vi "Periodic Tasks.vi"(8 "error in":errorcluster) -> ()   [LabVIEW 2015]
doc: "This VI runs in parallel to other tasks. It can contain as many user-defined periodic loops as you need. These can carry out PID or other sorts of timed response."
uses:
  <vilib>/Rock Robotics/WPI/Solenoid/WPI_SolenoidValue.ctl
  <vilib>/Rock Robotics/WPI/Utilities/WPI_GetSetVariantRefNum.vi
  Robot Global Data.vi
  <vilib>/Rock Robotics/WPI/Solenoid/WPI_SolenoidSetEnum.vi
  <vilib>/Rock Robotics/Network Tables/NT Write Boolean.vi
  <vilib>/Rock Robotics/Network Tables/NT Read Boolean.vi
  <vilib>/Rock Robotics/Network Tables/NT Read Number.vi
  <vilib>/addons/control/pid/pid.llb/PID (DBL).vi
  <vilib>/addons/control/pid/NI_PID_pid.lvlib
panel:
  out "Shoot Speed":dbl
  in  "Aiming Correction":dbl=-0.22
  out "Shoot Motor Output bottom 2":dbl
  out "Shoot Motor Output top 2":dbl
  out "Ball in Robot":bool
  out "Joystick Buttons":bool[](array[boolean])
  out "Joystick Axes":dbl[](array[numeric])
  out "RD before":bool
  out "RU before":bool
  out "R after":bool
  out "L after":bool
  out "LD before":bool
  out "LU before":bool
  out "Intake Mode":bool
  out "Low Mode":bool
  out "Shoot Sequence Position":dbl
  in  "Forklift Method":bool
  in  "Manual Shoot Speed":dbl=0.9
  out "Closed Loop Error":dbl
  out "Sensor Position":dbl
  in  "Expected position":dbl
  in  "Intake Speed":dbl=1.0
  out "Shoot Motor Output bottom":dbl
  out "Shoot Motor Output top":dbl
  in  "Aiming Speed":dbl(slide)=0.3 scale=0.0..1.0
  # "0 = Wait for trigger\n1 = Speed up and aim\n2 = Spin Rollers\n3 = Stop motors"
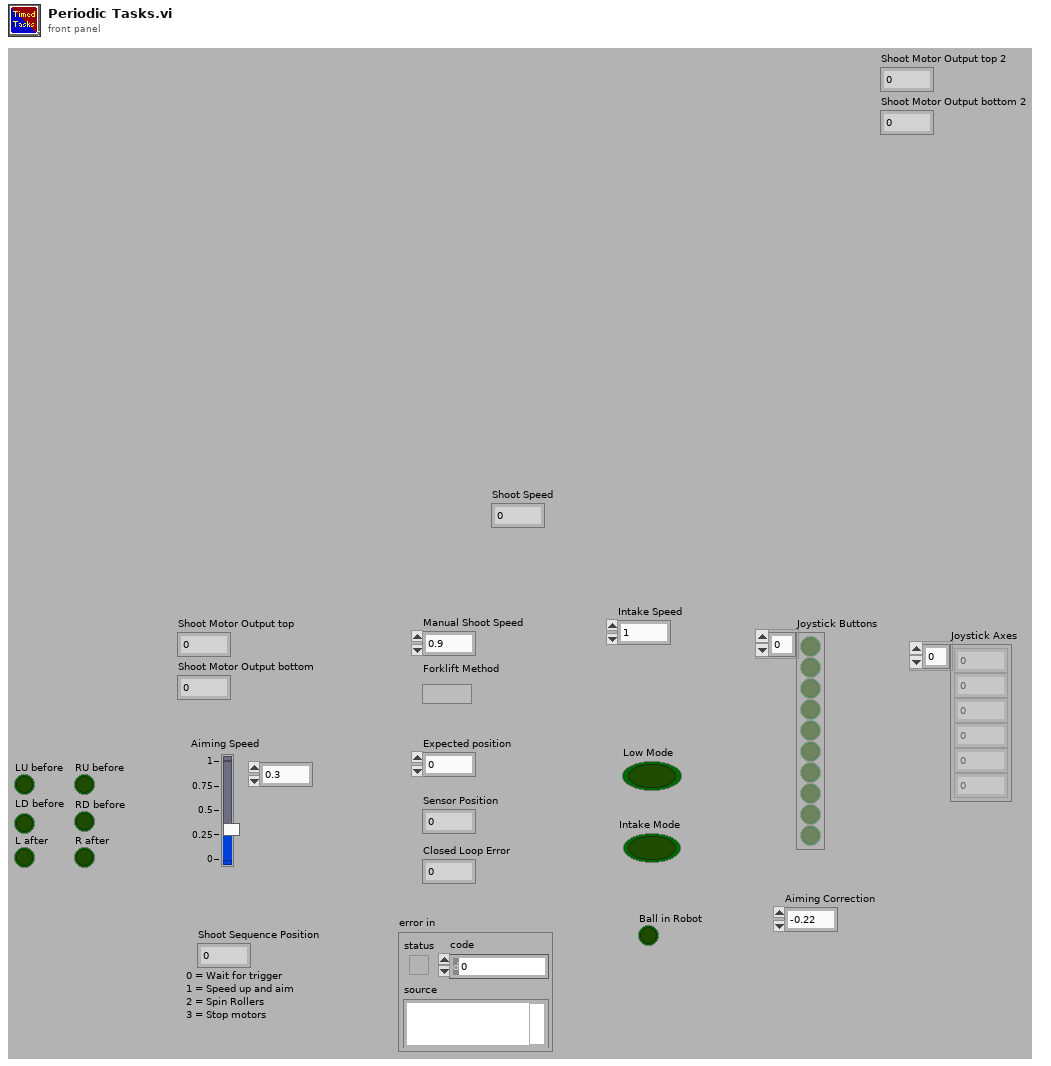
[diagram p1: front panel]
types:
  T1 = typedef "WPI_SolenoidDevRef.ctl" = cluster{"DevStatus":errorcluster, "Pneumatics Control Module":u8, "Forward Solenoid Channel":T2, "Reverse Solenoid Channel":T2}
  T2 = typedef "WPI_SolenoidChannel.ctl" = enum8{"Solenoid 0", "Solenoid 1", "Solenoid 2", "Solenoid 3", "Solenoid 4", "Solenoid 5", "Solenoid 6", "Solenoid 7", "Invalid"}
  T3 = typedef "WPI_JoystickDevRef.ctl" = cluster{"Device":T4}
  T4 = typedef "WPI_JoystickDeviceEnum.ctl" = enum16{"USB 0", "USB 1", "USB 2", "USB 3", "USB 4", "USB 5"}
  T5 = typedef "WPI_RobotDriveDevRef.ctl" = cluster{"DevStatus":errorcluster, "Motors[]":T6[], "Square Inputs":bool, "Max Output":dbl}
  T6 = typedef "WPI_MotorControlDeviceRef.ctl" = cluster{"DeviceStatus":errorcluster, "Type":T7, "PWM":cluster{"PWM Channel":T8, "DeadBand":T9}, "CAN":cluster{"Device Number":u8, "Control Mode":T10, "Semaphore":T11, "Max Vout":dbl, "TalonSRX Control Mode":T12}, "Invert":bool}
  T7 = typedef "WPI_MotorControlType.ctl" = enum16{"PWM", "CAN", "CANTalonSRX"}
  T8 = typedef "FPGA_DIOPWMChannel.ctl" = enum8{"PWM 0", "PWM 1", "PWM 2", "PWM 3", "PWM 4", "PWM 5", "PWM 6", "PWM 7", "PWM 8", "PWM 9", "PWM MXP 0", "PWM MXP 1", "PWM MXP 2", "PWM MXP 3", "PWM MXP 4", "PWM MXP 5", "PWM MXP 6", "PWM MXP 7", "PWM MXP 8", "PWM MXP 9", "Invalid"}
  T9 = typedef "WPI_PWMDeadband.ctl" = cluster{"Name":string, "maxPositivePwm":i32, "minPositivePwm":i32, "centerPwm":i32, "maxNegativePwm":i32, "minNegativePwm":i32, "angularRange":u16}
  T10 = typedef "WPI_CANJaguar_ControlMode.ctl" = enum8{"Percent VBus", "Current", "Speed", "Position", "Voltage"}
  T11 = typedef "Semaphore RefNum" = refnum<k1>
  T12 = typedef "WPI_CANTalonSRX_APIControlMode.ctl" = enum8{"Percent VBus", "Speed", "Position", "Slave", "Unchanged / Invalid", "Voltage Compensation", "Current", "Motion Profile"}
  T13 = typedef "WPI_I2CDevRef.ctl" = cluster{"DevStatus":errorcluster, "Device Address":u8, "Handle":i32, "I2C Bus":T14}
  T14 = typedef "i2c_bus.ctl" = enum16{"I2C On-Board", "I2C MXP", "Invalid"}
  T15 = typedef "WPI_DigitalInputDevRef.ctl" = cluster{"DevStatus":errorcluster, "DIO Channel":T16}
  T16 = typedef "FPGA_DIOChannel.ctl" = enum8{"DIO 0", "DIO 1", "DIO 2", "DIO 3", "DIO 4", "DIO 5", "DIO 6", "DIO 7", "DIO 8", "DIO 9", "DIO MXP 0", "DIO MXP 1", "DIO MXP 2", "DIO MXP 3", "DIO MXP 4", "DIO MXP 5", "DIO MXP 6", "DIO MXP 7", "DIO MXP 8", "DIO MXP 9", "DIO MXP 10", "DIO MXP 11", "DIO MXP 12", "DIO MXP 13", "DIO MXP 14", "DIO MXP 15", "Invalid"}
  T17 = cluster{"JoystickDevRef":T3, "RobotDriveDevRef":T5, "MotorControlDevRef":T6, "MotorControlDevRef":T6, "MotorControlDevRef":T6, "MotorControlDevRef":T6, "MotorControlDevRef":T6, "I2CDevRef":T13, "MotorControlDevRef":T6, "MotorControlDevRef":T6, "DigitalInputDevRef":T15, "SolenoidDevRef":T1, "SolenoidDevRef":T1, "SolenoidDevRef":T1}
  T18 = cluster{"Numeric":dbl, "Numeric":dbl, "Numeric":dbl}
  T19 = typedef "WPI_CANTalonSRX_GlobalStatus.ctl" = cluster{"Applied Throttle":dbl, "Module Enabled":bool, "CAN Error":errorcluster, "Closed Loop Error":dbl, "Forward Limit Switch Closed":bool, "Reverse Limit Switch Closed":bool, "Sensor Position":dbl, "Sensor Velocity":dbl, "Current":dbl, "Sticky Fault - Over Temp":bool, "Sticky Fault - Under Voltage":bool, "Sticky Fault - Forward Limit":bool, "Sticky Fault - Reverse Limit":bool, "Sticky Fault - Forward Soft Limit":bool, "Sticky Fault - Reverse Soft Limit":bool, "Brake is Enabled":bool, "Encoder Position":dbl, "Encoder Velocity":dbl, "Encoder Index Count":dbl, "Encoder A Pin State":bool, "Encoder B Pin State":bool, "Encoder Index Pin State":bool, "Analog In":dbl, "Analog In Velocity":dbl, "Temperature (C)":dbl, "Battery Voltage":dbl, "Control 5 Is Supported":bool, "Current Profile Slot Select":dbl, "Pos Div 8":bool, "Vel Div 4":bool, "Pulse Width Position":i32, "Pulse Width Velocity":i32, "Pulse Width Rise To Rise (us)":i32, "Pulse Width Rise To Fall (us)":i32, "Mot Prof Active Is Under Run":bool, "Mot Prof Active Has Under Run":bool, "Mot Prof Active Is Last":bool, "Mot Prof Active Velocity Only":bool, "Mot Prof Active Is Valid":bool, "Mot Prof Buffer Is Full":bool, "Mot Prof Active Profile Slot Select":i32, "Mot Prof NextID":i32, "Mot Prof Count":i32, "Mot Prof Active Velocity":dbl, "Mot Prof Active Position":dbl, "Mot Prof Output Enable":i32}
  T20 = typedef "WPI_SolenoidValue.ctl" = enum16{"Off", "On", "Forward", "Reverse"}
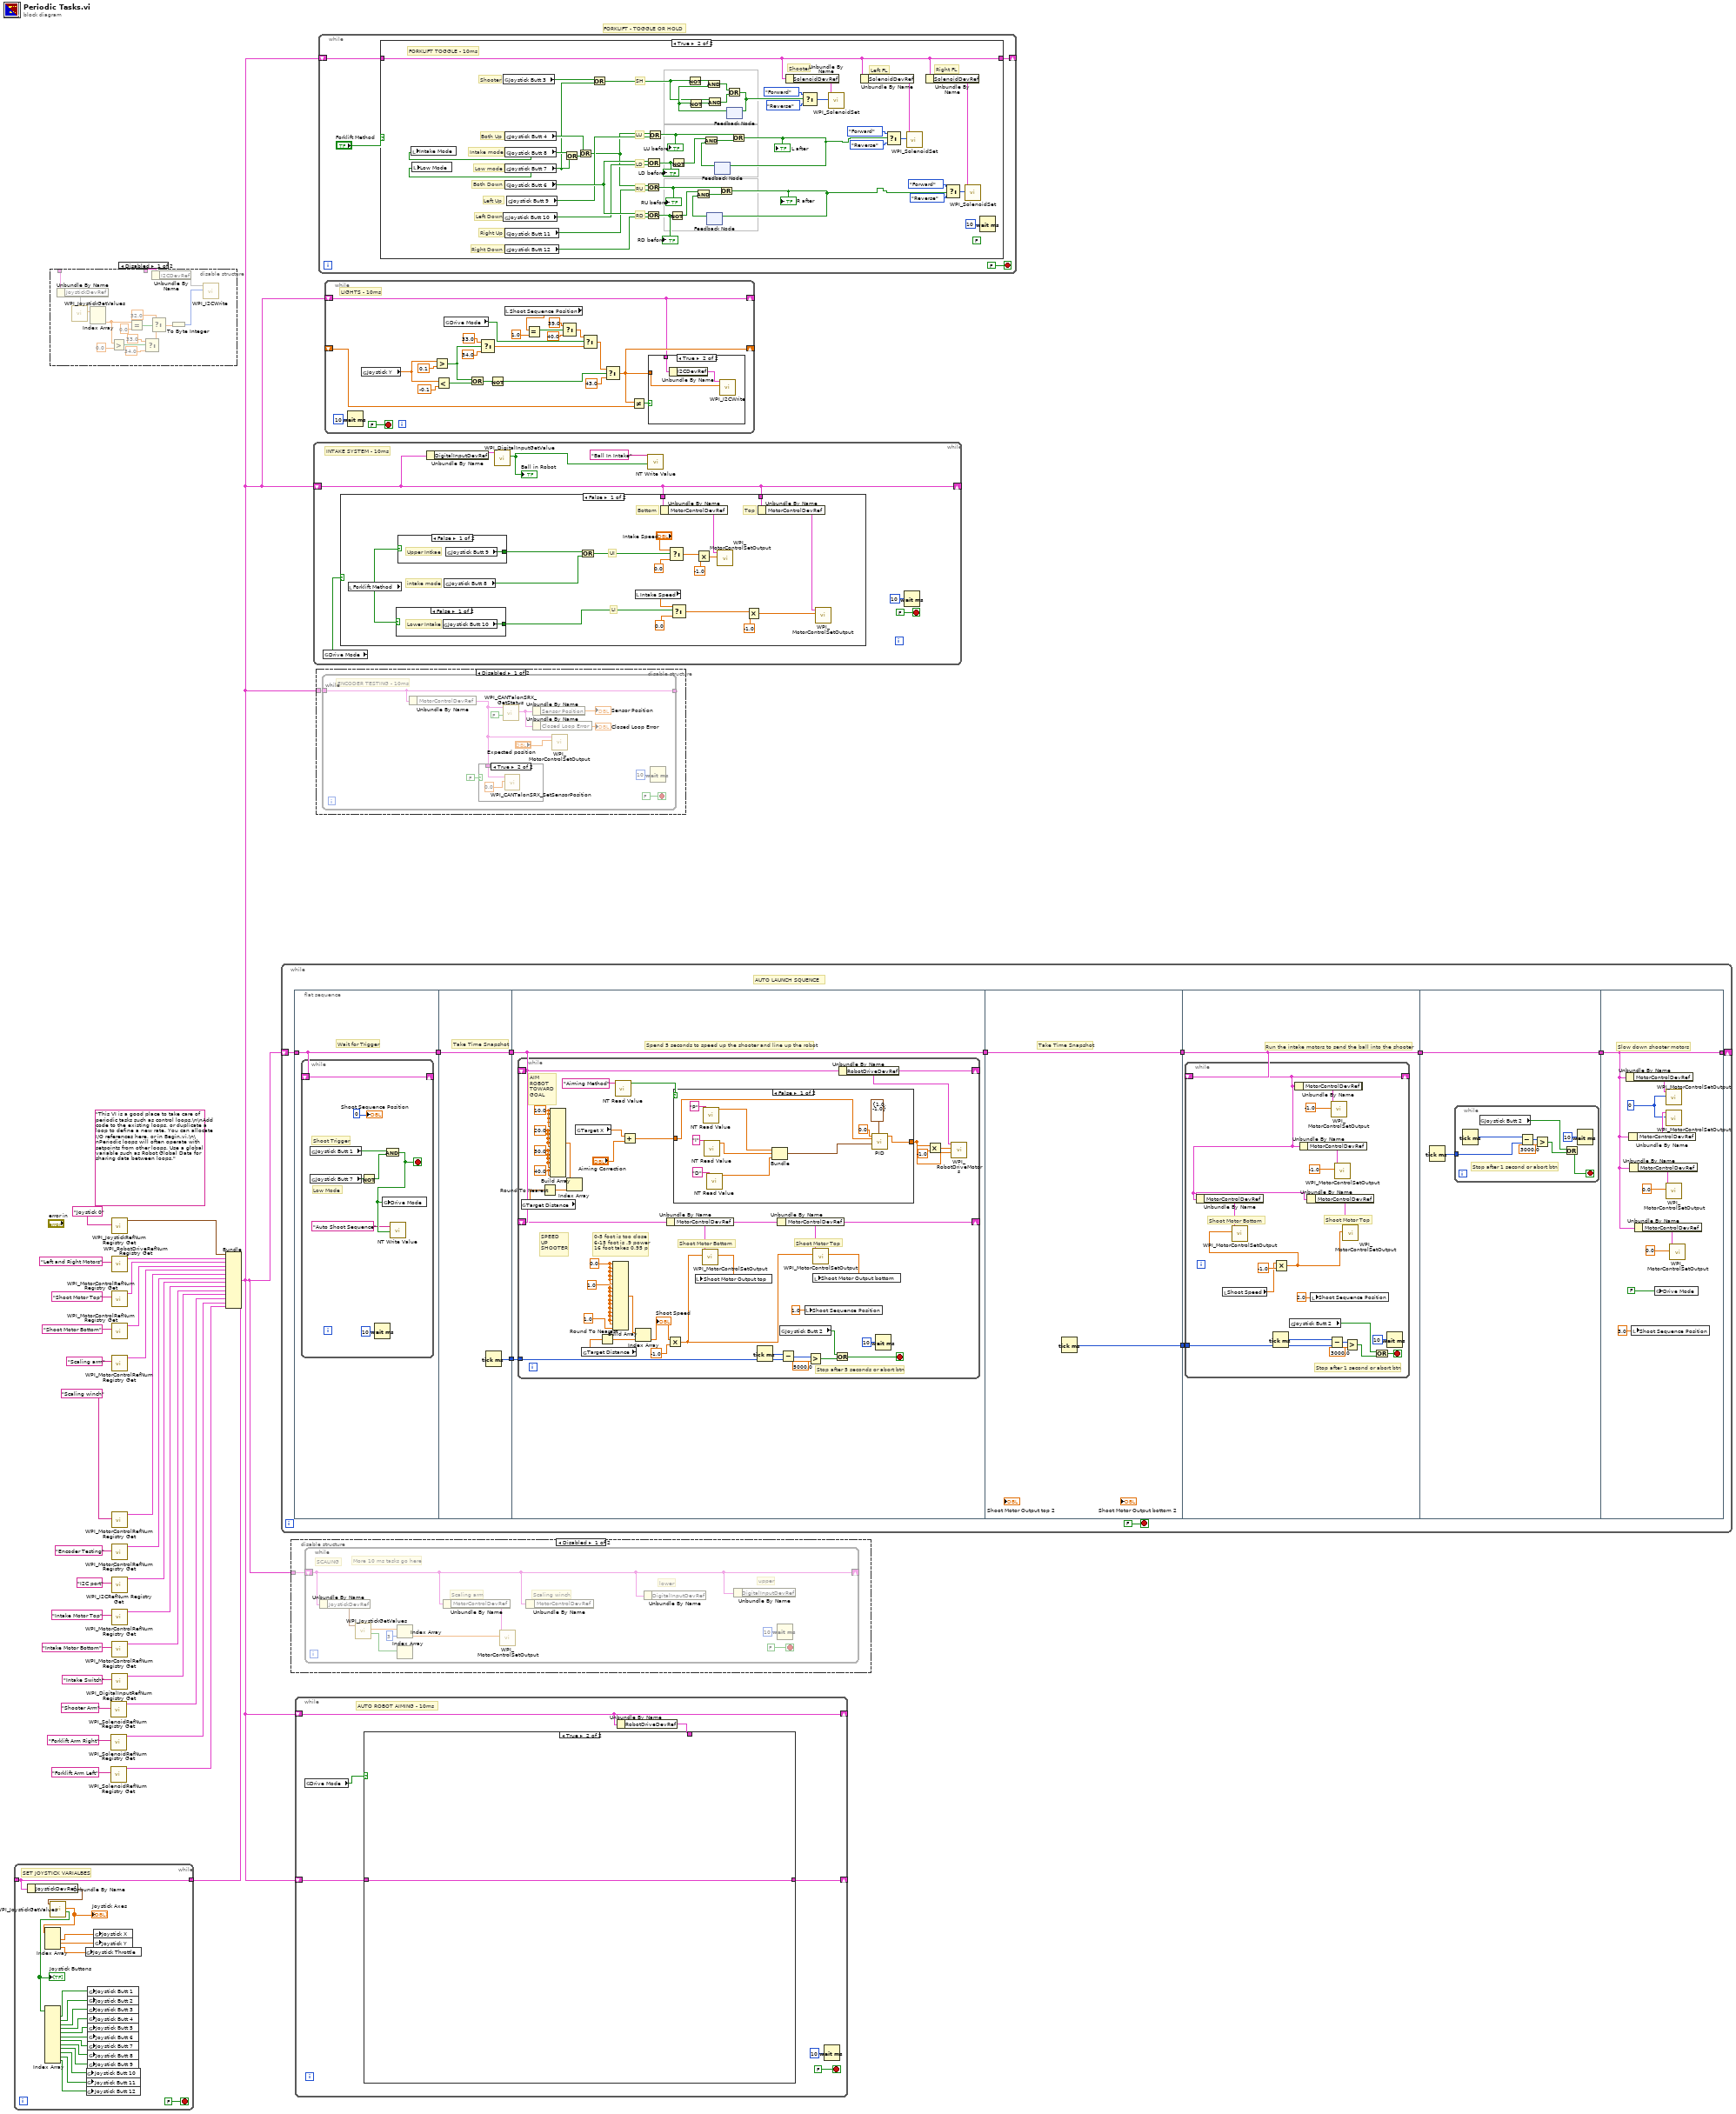
[diagram p0: block diagram]
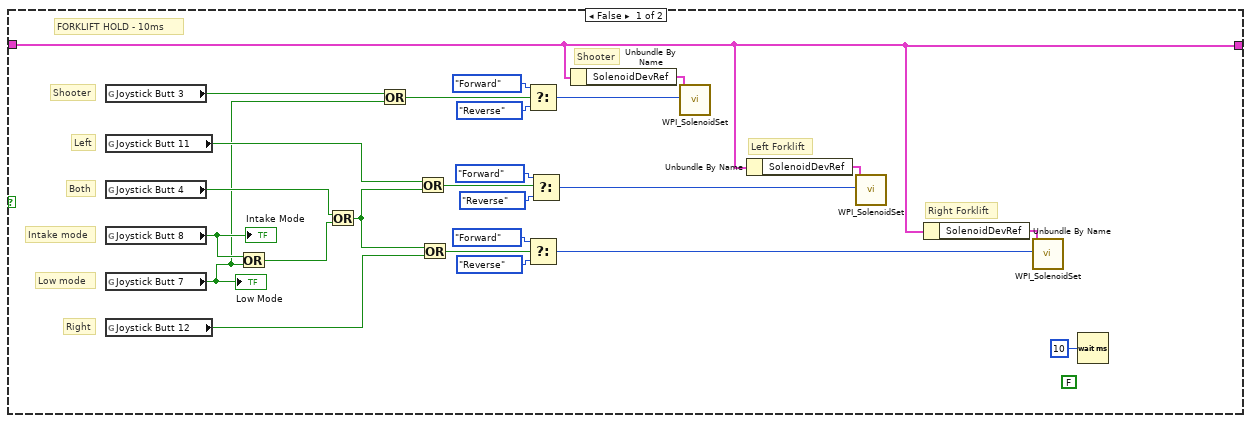
[diagram p2: hidden frame]
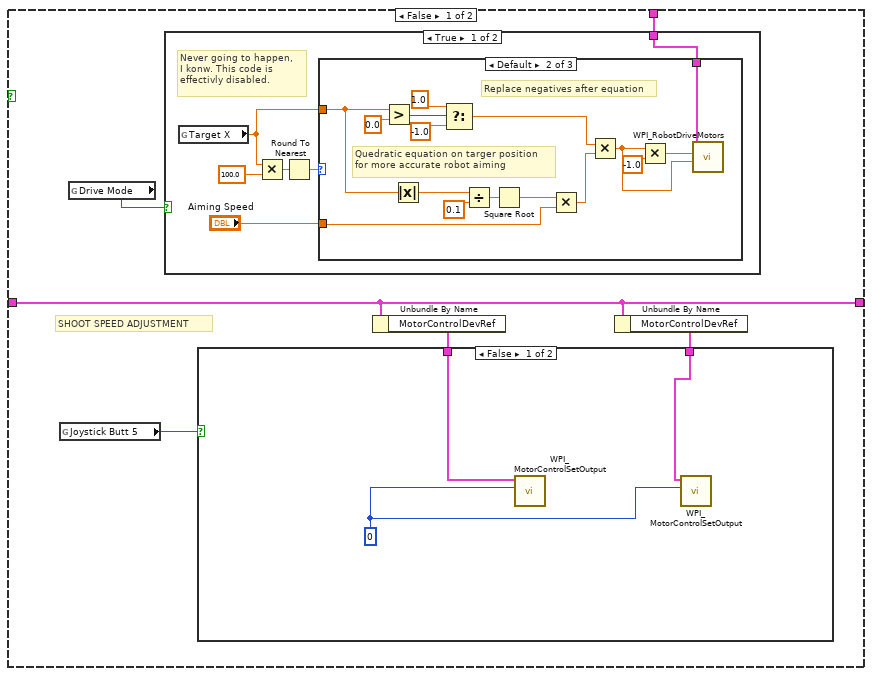
[diagram p6: hidden frame]
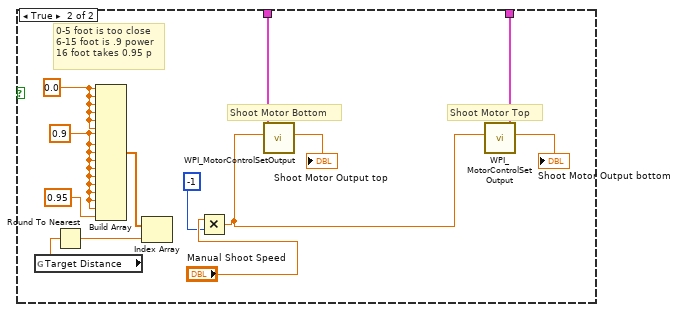
[diagram p7: hidden frame]
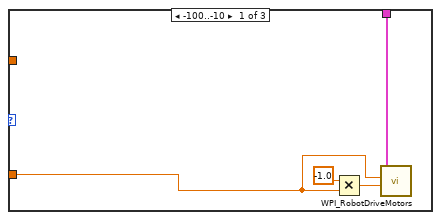
[diagram p8: hidden frame]
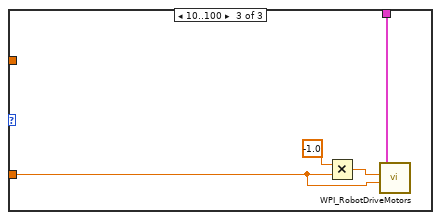
[diagram p9: hidden frame]
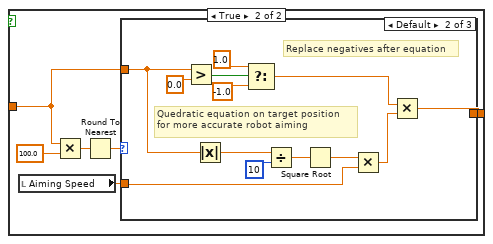
[diagram p11: hidden frame]
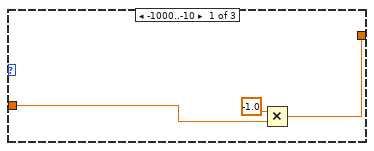
[diagram p12: hidden frame]
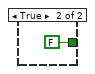
[diagram p15: hidden frame]
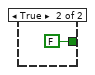
[diagram p16: hidden frame]
diagram:
  (unwired) "This VI is a good place to take care of periodic tasks such as control loops.\n\nAdd code to the existing loops, or duplicate a loop to define a new rate. You can allocate I/O references here, or in Begin.vi.\n\nPeriodic loops will often operate with setpoints from other loops. Use a global variable such as Robot Global Data for sharing data between loops."
  # "FORKLIFT - TOGGLE OR HOLD"
  n1 = disable-structure shown="Disabled" {
    disable-tunnel: _ -> [w44 _]
    disable-tunnel: _ -> [w40 _]
    frame Disabled {
      n2 = Unbundle By Name(w40) -> ("JoystickDevRef"=w42)
      n3 = call <vilib>:"WPI_JoystickGetValues.vi"("JoystickDevRef"=w42) -> ("Axes"=w43:dbl[])  [unwired: 6 in, 4 out]
      n4 = Index Array(array=w43) -> (element #2=w36:dbl)  [unwired: 2 in, 1 out]
      n5 = Greater?(x=w36, y=0.0) -> (0:w34:bool)
      n6 = Equal?(x=w36, y=0.0) -> (x = y?=w38:bool)
      n7 = Select(t=33.0, s=w34, f=34.0) -> (s? t:f=w37:dbl)
      n8 = Select(t=32.0, s=w38, f=w37) -> (s? t:f=w31:dbl)
      n9 = Unbundle By Name(w44) -> ("I2CDevRef"=w45)
      n10 = To Byte Integer(number=w31) -> (8bit integer=w30:i8)
      n11 = call <vilib>:"WPI_I2CWrite.vi"("I2CRegister"=w30, "I2CDevRef"=w45) -> ()  [unwired: 8 in, 2 out]
    }
    frame Enabled {
    }
  }
  n12 = call <vilib>:"WPI_SolenoidRefNum Registry Get.vi"("refnum name"="Shooter Arm") -> ("SolenoidDevRef"=w4:T1)  [unwired: 9 in, 1 out]
  n13 = call <vilib>:"WPI_SolenoidRefNum Registry Get.vi"("refnum name"="Forklift Arm Right") -> ("SolenoidDevRef"=w3:T1)  [unwired: 9 in, 1 out]
  n14 = call <vilib>:"WPI_SolenoidRefNum Registry Get.vi"("refnum name"="Forklift Arm Left") -> ("SolenoidDevRef"=w2:T1)  [unwired: 9 in, 1 out]
  n15 = call <vilib>:"WPI_JoystickRefNum Registry Get.vi"("refnum name"="Joystick 0") -> ("JoystickDevRef"=w27:T3)  [unwired: 1 in, 9 out]
  n16 = call <vilib>:"WPI_RobotDriveRefNum Registry Get.vi"("refnum name"="Left and Right Motors") -> ("RobotDriveDevRef"=w26:T5)  [unwired: 1 in, 9 out]
  n17 = call <vilib>:"WPI_MotorControlRefNum Registry Get.vi"("refnum name"="Shoot Motor Top") -> ("MotorControlDevRef"=w22:T6)  [unwired: 9 in, 1 out]
  n18 = call <vilib>:"WPI_MotorControlRefNum Registry Get.vi"("refnum name"="Shoot Motor Bottom") -> ("MotorControlDevRef"=w21:T6)  [unwired: 9 in, 1 out]
  n19 = call <vilib>:"WPI_MotorControlRefNum Registry Get.vi"("refnum name"="Scaling arm") -> ("MotorControlDevRef"=w20:T6)  [unwired: 9 in, 1 out]
  n20 = call <vilib>:"WPI_MotorControlRefNum Registry Get.vi"("refnum name"="Scaling winch") -> ("MotorControlDevRef"=w18:T6)  [unwired: 9 in, 1 out]
  n21 = call <vilib>:"WPI_MotorControlRefNum Registry Get.vi"("refnum name"="Encoder Testing") -> ("MotorControlDevRef"=w16:T6)  [unwired: 9 in, 1 out]
  n22 = call <vilib>:"WPI_I2CRefNum Registry Get.vi"("refnum name"="I2C port") -> ("I2CDevRef"=w15:T13)  [unwired: 9 in, 1 out]
  n23 = call <vilib>:"WPI_MotorControlRefNum Registry Get.vi"("refnum name"="Intake Motor Top") -> ("MotorControlDevRef"=w9:T6)  [unwired: 9 in, 1 out]
  n24 = call <vilib>:"WPI_MotorControlRefNum Registry Get.vi"("refnum name"="Intake Motor Bottom") -> ("MotorControlDevRef"=w8:T6)  [unwired: 9 in, 1 out]
  n25 = call <vilib>:"WPI_DigitalInputRefNum Registry Get.vi"("refnum name"="Intake Switch") -> ("DigitalInputDevRef"=w10:T15)  [unwired: 9 in, 1 out]
  n26 = Bundle("JoystickDevRef"=w27, "RobotDriveDevRef"=w26, "MotorControlDevRef"=w22, "MotorControlDevRef"=w21, "MotorControlDevRef"=w20, "MotorControlDevRef"=w18, "MotorControlDevRef"=w16, "I2CDevRef"=w15, "MotorControlDevRef"=w9, "MotorControlDevRef"=w8, "DigitalInputDevRef"=w10, "SolenoidDevRef"=w4, "SolenoidDevRef"=w3, "SolenoidDevRef"=w2) -> (w1:T17)  [unwired: 1 out]
  n27 = while {
    tunnel: [w65] -> _
    tunnel: w1 -> [w65]
    stop <- FALSE stop-if-true
    # "SET JOYSTICK VARIALBES"
    n28 = Unbundle By Name(w65) -> ("JoystickDevRef"=w64:T3)
    n29 = call <vilib>:"WPI_JoystickGetValues.vi"("JoystickDevRef"=w64) -> ("Buttons"=w62:bool[], "Axes"=w63:dbl[])  [unwired: 6 in, 3 out]
    "Joystick Axes" <- w63
    "Joystick Buttons" <- w62
    n30 = Index Array(array=w63) -> (element #1=w52:dbl, element #2=w51:dbl, element #3=w50:dbl)  [unwired: 3 in]
    n31 = Index Array(array=w62) -> (element #1=w48:bool, element #2=w61:bool, element #3=w47:bool, element #4=w60:bool, element #5=w46:bool, element #6=w59:bool, element #7=w58:bool, element #8=w57:bool, element #9=w56:bool, element #10=w55:bool, element #11=w54:bool, element #12=w53:bool)  [unwired: 12 in]
    n32 = global write "Robot Global Data.vi" "Joystick Throttle"(w50) -> ()
    n33 = global write "Robot Global Data.vi" "Joystick Butt 10"(w55) -> ()
    n34 = global write "Robot Global Data.vi" "Joystick Butt 11"(w54) -> ()
    n35 = global write "Robot Global Data.vi" "Joystick Butt 12"(w53) -> ()
    n36 = global write "Robot Global Data.vi" "Joystick Butt 1"(w48) -> ()
    n37 = global write "Robot Global Data.vi" "Joystick Butt 2"(w61) -> ()
    n38 = global write "Robot Global Data.vi" "Joystick Butt 3"(w47) -> ()
    n39 = global write "Robot Global Data.vi" "Joystick Butt 4"(w60) -> ()
    n40 = global write "Robot Global Data.vi" "Joystick Butt 5"(w46) -> ()
    n41 = global write "Robot Global Data.vi" "Joystick Butt 6"(w59) -> ()
    n42 = global write "Robot Global Data.vi" "Joystick Butt 7"(w58) -> ()
    n43 = global write "Robot Global Data.vi" "Joystick Butt 8"(w57) -> ()
    n44 = global write "Robot Global Data.vi" "Joystick Butt 9"(w56) -> ()
    n45 = global write "Robot Global Data.vi" "Joystick X"(w52) -> ()
    n46 = global write "Robot Global Data.vi" "Joystick Y"(w51) -> ()
  }
  n47 = while {
    shift-right: [w75] -> _
    shift-left: w1 -> [w76]
    stop <- FALSE stop-if-true
    # "AUTO LAUNCH SQUENCE"
    n48 = flat-sequence {
      tunnel: w76 -> [w77]
      tunnel: [w77] -> w73
      tunnel: w73 -> [w87]
      tunnel: [w87] -> w72
      tunnel: [w86] -> w69
      tunnel: w72 -> [w89]
      tunnel: [w89] -> w71
      tunnel: w69 -> [w88]
      tunnel: w71 -> [w165]
      tunnel: [w165] -> w70
      tunnel: [w164] -> w68
      tunnel: [w167] -> w67
      tunnel: w70 -> [w167]
      tunnel: w68 -> [w166]
      tunnel: w67 -> [w188]
      tunnel: [w188] -> w66
      tunnel: [w199] -> w75
      tunnel: w66 -> [w199]
      frame #0 {
        # "Wait for Trigger"
        n49 = while {
          shift-right: [w83] -> _
          shift-left: w77 -> [w83]
          stop <- w79 stop-if-true
          # "Shoot Trigger"
          # "Low Mode"
          n50 = global read "Robot Global Data.vi" "Joystick Butt 1"() -> (w80:bool)
          n51 = global read "Robot Global Data.vi" "Joystick Butt 7"() -> (w82:bool)
          n52 = Not(x=w82) -> (.not. x?=w81:bool)
          n53 = Wait (ms)(milliseconds to wait=u32 10) -> ()  [unwired: 1 out]
          n54 = And(x=w80, y=w81) -> (x .and. y?=w79:bool)
          n55 = global write "Robot Global Data.vi" "Drive Mode"(w79) -> ()
          n56 = call-poly <vilib>:"NT Write Value.vi"("Boolean"=w79, "Name"="Auto Shoot Sequence") -> ()  [unwired: 9 in, 1 out]
          "Shoot Sequence Position" <- 0
        }
      }
      frame #1 {
        # "Take Time Snapshot"
        n57 = Tick Count (ms)() -> (millisecond timer value=w86:u32)
      }
      frame #2 {
        # "Spend 5 seconds to speed up the shooter and line up the robot"
        n58 = while {
          shift-right: [w119] -> _
          shift-left: w89 -> [w119]
          shift-right: [w113] -> _
          shift-left: w89 -> [w113]
          tunnel: w88 -> [w100]
          stop <- w117 stop-if-true
          w104 = 40.0 ("element")
          w105 = 30.0 ("element")
          w106 = 20.0 ("element")
          w107 = 10.0 ("element")
          w123 = 1.0
          w124 = 0.0
          # "SPEED\nUP \nSHOOTER"
          # "AIM\nROBOT\nTOWARD\nGOAL"
          # "0-5 foot is too close\n6-15 foot is .9 power\n16 foot takes 0.95 p"
          # "Shoot Motor Bottom"
          # "Shoot Motor Top"
          # "Stop after 5 seconds or abort btn"
          n59 = global read "Robot Global Data.vi" "Target Distance"() -> (w102:dbl)
          n60 = Round To Nearest(number=w102) -> (nearest integer value=w103:dbl)
          n61 = Build Array(w107, w107, w107, w107, w107, w106, w106, w106, w106, w106, w105, w105, w105, w105, w105, w104, w104) -> (w108:dbl[])
          n62 = Index Array(array=w108, index=w103) -> ()  [unwired: 1 out]
          n63 = global read "Robot Global Data.vi" "Target X"() -> (w98:dbl)
          n64 = global read "Robot Global Data.vi" "Target Distance"() -> (w128:dbl)
          n65 = Round To Nearest(number=w128) -> (nearest integer value=w126:dbl)
          n66 = Build Array(w124, w124, w124, w124, w124, w124, w123, w123, w123, w123, w123, w123, w123, w123, w123, w123, 1.0) -> (w127:dbl[])
          n67 = call-poly <vilib>:"NT Read Value.vi"("Name"="Aiming Method") -> ("Boolean"=w91:bool)  [unwired: 9 in, 1 out]
          n68 = Add(x=w98, y="Aiming Correction") -> (x+y=w97:dbl)
          n69 = Index Array(array=w127, index=w126) -> (element=w116:dbl)
          "Shoot Speed" <- w116
          n70 = Unbundle By Name(w113) -> ("MotorControlDevRef"=w122:T6)
          n71 = Multiply(x=w116, y=-1.0 ("f")) -> (x*y=w115:dbl)
          n72 = case shown="False" w91 {
            tunnel: w97 -> [w131 w142]
            tunnel: [w133 w141] -> w93
            frame False {
              n73 = call-poly <vilib>:"NT Read Value.vi"("Name"="P") -> ("Numeric"=w137:dbl)  [unwired: 9 in, 1 out]
              n74 = call-poly <vilib>:"NT Read Value.vi"("Name"="I") -> ("Numeric"=w136:dbl)  [unwired: 9 in, 1 out]
              n75 = call-poly <vilib>:"NT Read Value.vi"("Name"="D") -> ("Numeric"=w135:dbl)  [unwired: 9 in, 1 out]
              n76 = Bundle("Numeric"=w137, "Numeric"=w136, "Numeric"=w135) -> (w134:T18)  [unwired: 1 in]
              n77 = call-poly <vilib>:"PID.vi"("output range"=cluster{"output high":dbl, "output low":dbl} {"output high"=1.0, "output low"=-1.0}, "PID gains"=w134, "process variable"=w131, "setpoint"=0.0) -> ("output"=w133:dbl)  [unwired: 6 in, 1 out]
            }
            frame True {
              n78 = local read "Aiming Speed"() -> (w144:dbl)
              n79 = Multiply(x=w142, y=100.0) -> (x*y=w143:dbl)
              n80 = Round To Nearest(number=w143) -> (nearest integer value=w146:dbl)
              n81 = case shown="Default" w146 {
                tunnel: w144 -> [w148 w161 w163]
                tunnel: w142 -> [_ w157 _]
                tunnel: [w147 w150 w163] -> w141
                frame -1000..-10 {
                  n82 = Multiply(x=-1.0 ("y"), y=w148) -> (x*y=w147:dbl)
                }
                frame Default {
                  # "Replace negatives after equation"
                  # "Quedratic equation on target position\nfor more accurate robot aiming"
                  n83 = Greater?(x=w157, y=0.0) -> (0:w159:bool)
                  n84 = Absolute Value(x=w157) -> (abs(x)=w156:dbl)
                  n85 = Select(t=1.0, s=w159, f=-1.0) -> (s? t:f=w158:dbl)
                  n86 = Divide(x=w156, y=10) -> (x/y=w152:dbl)
                  n87 = Square Root(x=w152) -> (sqrt(x)=w151:dbl)
                  n88 = Multiply(x=w151, y=w161) -> (x*y=w153:dbl)
                  n89 = Multiply(x=w158, y=w153) -> (x*y=w150:dbl)
                }
                frame 10..1000 {
                }
              }
            }
          }
          n90 = call <vilib>:"WPI_MotorControlSetOutput.vi"("Output"=w115, "MotorControlDevRef"=w122) -> ("Motor Output"=w109:dbl)  [unwired: 7 in, 2 out]
          n91 = local write "Shoot Motor Output top"(w109) -> ()
          n92 = Tick Count (ms)() -> (millisecond timer value=w99:u32)
          n93 = Unbundle By Name(w113) -> ("MotorControlDevRef"=w121:T6)
          n94 = global read "Robot Global Data.vi" "Joystick Butt 2"() -> (w112:bool)
          n95 = Subtract(x=w99, y=w100) -> (x-y=w101:u32)
          n96 = local write "Shoot Sequence Position"(1.0 ("Shoot Sequence Position")) -> ()
          n97 = Greater?(x=w101, y=5000.0) -> (0:w118:bool)
          n98 = call <vilib>:"WPI_MotorControlSetOutput.vi"("Output"=w115, "MotorControlDevRef"=w121) -> ("Motor Output"=w110:dbl)  [unwired: 7 in, 2 out]
          n99 = local write "Shoot Motor Output bottom"(w110) -> ()
          n100 = Or(x=w112, y=w118) -> (x .or. y?=w117:bool)
          n101 = Unbundle By Name(w119) -> ("RobotDriveDevRef"=w92:T5)
          n102 = Wait (ms)(milliseconds to wait=u32 10) -> ()  [unwired: 1 out]
          n103 = Multiply(x=w93, y=-1.0) -> (x*y=w94:dbl)
          n104 = call <vilib>:"WPI_RobotDriveMotors.vi"("RightSpeed"=w93, "LeftSpeed"=w94, "RobotDriveDevRef"=w92) -> ()  [unwired: 6 in, 3 out]
        }
      }
      frame #3 {
        # "Take Time Snapshot"
        n105 = Tick Count (ms)() -> (millisecond timer value=w164:u32)
      }
      frame #4 {
        # "Run the intake motors to send the ball into the shooter"
        n106 = while {
          shift-right: [w171] -> _
          shift-left: w167 -> [w171]
          tunnel: w166 -> [w175]
          stop <- w181 stop-if-true
          # "Shoot Motor Bottom"
          # "Shoot Motor Top"
          # "Stop after 1 second or abort btn"
          n107 = Unbundle By Name(w171) -> ("MotorControlDevRef"=w172:T6)
          n108 = local read "Shoot Speed"() -> (w169:dbl)
          n109 = Tick Count (ms)() -> (millisecond timer value=w174:u32)
          n110 = Multiply(x=w169, y=-1.0) -> (x*y=w168:dbl)
          n111 = call <vilib>:"WPI_MotorControlSetOutput.vi"("Output"=w168, "MotorControlDevRef"=w172) -> ()  [unwired: 7 in, 3 out]
          n112 = global read "Robot Global Data.vi" "Joystick Butt 2"() -> (w180:bool)
          n113 = Unbundle By Name(w171) -> ("MotorControlDevRef"=w182:T6)
          n114 = Unbundle By Name(w171) -> ("MotorControlDevRef"=w186:T6)
          n115 = Unbundle By Name(w171) -> ("MotorControlDevRef"=w173:T6)
          n116 = local write "Shoot Sequence Position"(2.0 ("Shoot Sequence Position")) -> ()
          n117 = Subtract(x=w174, y=w175) -> (x-y=w178:u32)
          n118 = call <vilib>:"WPI_MotorControlSetOutput.vi"("Output"=-1.0, "MotorControlDevRef"=w182) -> ()  [unwired: 7 in, 3 out]
          n119 = call <vilib>:"WPI_MotorControlSetOutput.vi"("Output"=-1.0, "MotorControlDevRef"=w186) -> ()  [unwired: 7 in, 3 out]
          n120 = call <vilib>:"WPI_MotorControlSetOutput.vi"("Output"=w168, "MotorControlDevRef"=w173) -> ()  [unwired: 7 in, 3 out]
          n121 = Greater?(x=w178, y=3000.0) -> (0:w176:bool)
          n122 = Or(x=w180, y=w176) -> (x .or. y?=w181:bool)
          n123 = Wait (ms)(milliseconds to wait=u32 10) -> ()  [unwired: 1 out]
        }
      }
      frame #5 {
        n124 = Tick Count (ms)() -> (millisecond timer value=w187:u32)
        n125 = while {
          tunnel: w187 -> [w189]
          stop <- w190 stop-if-true
          # "Stop after 1 second or abort btn"
          n126 = Tick Count (ms)() -> (millisecond timer value=w191:u32)
          n127 = global read "Robot Global Data.vi" "Joystick Butt 2"() -> (w195:bool)
          n128 = Subtract(x=w191, y=w189) -> (x-y=w194:u32)
          n129 = Greater?(x=w194, y=3000.0) -> (0:w192:bool)
          n130 = Or(x=w195, y=w192) -> (x .or. y?=w190:bool)
          n131 = Wait (ms)(milliseconds to wait=u32 10) -> ()  [unwired: 1 out]
        }
      }
      frame #6 {
        w204 = 0
        # "Slow down shooter motors"
        n132 = Unbundle By Name(w199) -> ("MotorControlDevRef"=w206:T6)
        n133 = Unbundle By Name(w199) -> ("MotorControlDevRef"=w205:T6)
        n134 = Unbundle By Name(w199) -> ("MotorControlDevRef"=w200:T6)
        n135 = local write "Shoot Sequence Position"(3.0 ("Shoot Sequence Position")) -> ()
        n136 = Unbundle By Name(w199) -> ("MotorControlDevRef"=w203:T6)
        n137 = global write "Robot Global Data.vi" "Drive Mode"(FALSE ("Drive Mode")) -> ()
        n138 = call <vilib>:"WPI_MotorControlSetOutput.vi"("Output"=w204, "MotorControlDevRef"=w206) -> ()  [unwired: 7 in, 3 out]
        n139 = call <vilib>:"WPI_MotorControlSetOutput.vi"("Output"=w204, "MotorControlDevRef"=w205) -> ()  [unwired: 7 in, 3 out]
        n140 = call <vilib>:"WPI_MotorControlSetOutput.vi"("Output"=0.0, "MotorControlDevRef"=w200) -> ()  [unwired: 7 in, 3 out]
        n141 = call <vilib>:"WPI_MotorControlSetOutput.vi"("Output"=0.0, "MotorControlDevRef"=w203) -> ()  [unwired: 7 in, 3 out]
      }
    }
  }
  n142 = disable-structure shown="Disabled" {
    disable-tunnel: w1 -> [w207 _]
    frame Disabled {
      n143 = while {
        shift-right: [w208] -> _
        shift-left: w207 -> [w208]
        stop <- FALSE stop-if-true
        # "upper"
        # "lower"
        # "Scaling arm"
        # "Scaling winch"
        # "SCALING"
        # "More 10 ms tasks go here"
        n144 = Unbundle By Name(w208) -> ("JoystickDevRef"=w214:T3)
        n145 = call <vilib>:"WPI_JoystickGetValues.vi"("JoystickDevRef"=w214) -> ("Buttons"=w209:bool[], "Axes"=w212:dbl[])  [unwired: 6 in, 3 out]
        n146 = Index Array(array=w212, index=3) -> (element=w210:dbl)
        n147 = Index Array(array=w209) -> ()  [unwired: 1 in, 1 out]
        n148 = Unbundle By Name(w208) -> ("MotorControlDevRef"=w211:T6)
        n149 = call <vilib>:"WPI_MotorControlSetOutput.vi"("Output"=w210, "MotorControlDevRef"=w211) -> ()  [unwired: 7 in, 3 out]
        n150 = Unbundle By Name(w208) -> ()  [unwired: 1 out]
        n151 = Unbundle By Name(w208) -> ()  [unwired: 1 out]
        n152 = Unbundle By Name(w208) -> ()  [unwired: 1 out]
        n153 = Wait (ms)(milliseconds to wait=u32 10) -> ()  [unwired: 1 out]
      }
    }
    frame Enabled {
    }
  }
  n154 = while {
    shift-right: [w221] -> _
    shift-left: w1 -> [w221]
    shift-right: [w219] -> _
    shift-left: w1 -> [w220]
    stop <- FALSE stop-if-true
    # "AUTO ROBOT AIMING - 10ms"
    n155 = global read "Robot Global Data.vi" "Drive Mode"() -> (w217:bool)
    n156 = Unbundle By Name(w221) -> ("RobotDriveDevRef"=w218:T5)
    n157 = case shown="True" w217 {
      tunnel: w220 -> [w226 w276]
      tunnel: [w226 w276] -> w219
      tunnel: w218 -> [w225 _]
      frame False {
        # "SHOOT SPEED ADJUSTMENT"
        n158 = global read "Robot Global Data.vi" "Joystick Butt 5"() -> (w224:bool)
        n159 = global read "Robot Global Data.vi" "Drive Mode"() -> (w227:bool)
        n160 = case shown="True" w227 {
          tunnel: w225 -> [w246 _]
          frame True {
            # "Never going to happen,\nI konw. This code is \neffectivly disabled."
            n161 = global read "Robot Global Data.vi" "Target X"() -> (w250:dbl)
            n162 = Multiply(x=w250, y=100.0) -> (x*y=w251:dbl)
            n163 = Round To Nearest(number=w251) -> (nearest integer value=w248:dbl)
            n164 = case shown="Default" w248 {
              tunnel: w246 -> [w255 w270 w274]
              tunnel: "Aiming Speed" -> [w252 w267 w272]
              tunnel: w250 -> [_ w262 _]
              frame -100..-10 {
                n165 = Multiply(x=-1.0 ("y"), y=w252) -> (x*y=w253:dbl)
                n166 = call <vilib>:"WPI_RobotDriveMotors.vi"("RightSpeed"=w253, "LeftSpeed"=w252, "RobotDriveDevRef"=w255) -> ()  [unwired: 6 in, 3 out]
              }
              frame Default {
                # "Replace negatives after equation"
                # "Quedratic equation on targer position\nfor more accurate robot aiming"
                n167 = Greater?(x=w262, y=0.0) -> (0:w264:bool)
                n168 = Absolute Value(x=w262) -> (abs(x)=w261:dbl)
                n169 = Select(t=1.0, s=w264, f=-1.0) -> (s? t:f=w263:dbl)
                n170 = Divide(x=w261, y=0.1) -> (x/y=w268:dbl)
                n171 = Square Root(x=w268) -> (sqrt(x)=w266:dbl)
                n172 = Multiply(x=w266, y=w267) -> (x*y=w258:dbl)
                n173 = Multiply(x=w263, y=w258) -> (x*y=w256:dbl)
                n174 = Multiply(x=w256, y=-1.0) -> (x*y=w257:dbl)
                n175 = call <vilib>:"WPI_RobotDriveMotors.vi"("RightSpeed"=w256, "LeftSpeed"=w257, "RobotDriveDevRef"=w270) -> ()  [unwired: 6 in, 3 out]
              }
              frame 10..100 {
                n176 = Multiply(x=-1.0 ("y"), y=w272) -> (x*y=w273:dbl)
                n177 = call <vilib>:"WPI_RobotDriveMotors.vi"("RightSpeed"=w272, "LeftSpeed"=w273, "RobotDriveDevRef"=w274) -> ()  [unwired: 6 in, 3 out]
              }
            }
          }
          frame False {
          }
        }
        n178 = Unbundle By Name(w226) -> ("MotorControlDevRef"=w228:T6)
        n179 = Unbundle By Name(w226) -> ("MotorControlDevRef"=w229:T6)
        n180 = case shown="False" w224 {
          tunnel: w228 -> [w231 w242]
          tunnel: w229 -> [w232 w241]
          frame False {
            w230 = 0
            n181 = call <vilib>:"WPI_MotorControlSetOutput.vi"("Output"=w230, "MotorControlDevRef"=w231) -> ()  [unwired: 7 in, 3 out]
            n182 = call <vilib>:"WPI_MotorControlSetOutput.vi"("Output"=w230, "MotorControlDevRef"=w232) -> ()  [unwired: 7 in, 3 out]
          }
          frame True {
            w236 = 0.9
            w237 = 0.0
            # "0-5 foot is too close\n6-15 foot is .9 power\n16 foot takes 0.95 p"
            # "Shoot Motor Top"
            # "Shoot Motor Bottom"
            n183 = global read "Robot Global Data.vi" "Target Distance"() -> (w245:dbl)
            n184 = Round To Nearest(number=w245) -> (nearest integer value=w243:dbl)
            n185 = Build Array(w237, w237, w237, w237, w237, w237, w236, w236, w236, w236, w236, w236, w236, w236, w236, w236, 0.95) -> (w244:dbl[])
            n186 = Index Array(array=w244, index=w243) -> ()  [unwired: 1 out]
            n187 = Multiply(x="Manual Shoot Speed", y=-1) -> (x*y=w235:dbl)
            n188 = call <vilib>:"WPI_MotorControlSetOutput.vi"("Output"=w235, "MotorControlDevRef"=w242) -> ("Motor Output"=→"Shoot Motor Output top":dbl)  [unwired: 7 in, 2 out]
            n189 = call <vilib>:"WPI_MotorControlSetOutput.vi"("Output"=w235, "MotorControlDevRef"=w241) -> ("Motor Output"=→"Shoot Motor Output bottom":dbl)  [unwired: 7 in, 2 out]
          }
        }
      }
      frame True {
      }
    }
    n190 = Wait (ms)(milliseconds to wait=u32 10) -> ()  [unwired: 1 out]
  }
  n191 = while {
    shift-right: [w279] -> _
    shift-left: w1 -> [w279]
    stop <- FALSE stop-if-true
    # "INTAKE SYSTEM - 10ms"
    n192 = global read "Robot Global Data.vi" "Drive Mode"() -> (w281:bool)
    n193 = case shown="False" w281 {
      tunnel: w279 -> [w300 _]
      tunnel: w279 -> [w299 _]
      frame False {
        # "UI"
        # "LI"
        # "Bottom"
        # "Top"
        # "intake mode"
        n194 = local read "Forklift Method"() -> (w294:bool)
        n195 = case shown="False" w294 {
          tunnel: [w305 FALSE ("Joystick Butt 9")] -> w287
          frame False {
            # "Lower Intake"
            n196 = global read "Robot Global Data.vi" "Joystick Butt 10"() -> (w305:bool)
          }
          frame True {
          }
        }
        n197 = case shown="False" w294 {
          tunnel: [w303 FALSE ("Joystick Butt 10")] -> w286
          frame False {
            # "Upper Intkae"
            n198 = global read "Robot Global Data.vi" "Joystick Butt 9"() -> (w303:bool)
          }
          frame True {
          }
        }
        n199 = global read "Robot Global Data.vi" "Joystick Butt 8"() -> (w284:bool)
        n200 = Or(x=w286, y=w284) -> (x .or. y?=w285:bool)
        n201 = local read "Intake Speed"() -> (w297:dbl)
        n202 = Unbundle By Name(w299) -> ("MotorControlDevRef"=w301:T6)
        n203 = Select(t="Intake Speed", s=w285, f=0.0) -> (s? t:f=w291:dbl)
        n204 = Select(t=w297, s=w287, f=0.0) -> (s? t:f=w290:dbl)
        n205 = Multiply(x=w291, y=-1.0) -> (x*y=w292:dbl)
        n206 = call <vilib>:"WPI_MotorControlSetOutput.vi"("Output"=w292, "MotorControlDevRef"=w301) -> ()  [unwired: 7 in, 3 out]
        n207 = Multiply(x=w290, y=-1.0) -> (x*y=w288:dbl)
        n208 = Unbundle By Name(w300) -> ("MotorControlDevRef"=w302:T6)
        n209 = call <vilib>:"WPI_MotorControlSetOutput.vi"("Output"=w288, "MotorControlDevRef"=w302) -> ()  [unwired: 7 in, 3 out]
      }
      frame True {
      }
    }
    n210 = Unbundle By Name(w279) -> ("DigitalInputDevRef"=w280:T15)
    n211 = call <vilib>:"WPI_DigitalInputGetValue.vi"("DigitalInputDevRef"=w280) -> ("Value"=w278:bool)  [unwired: 8 in, 2 out]
    "Ball in Robot" <- w278
    n212 = call-poly <vilib>:"NT Write Value.vi"("Boolean"=w278, "Name"="Ball In Intake") -> ()  [unwired: 9 in, 1 out]
    n213 = Wait (ms)(milliseconds to wait=u32 10) -> ()  [unwired: 1 out]
  }
  n214 = disable-structure shown="Disabled" {
    disable-tunnel: w1 -> [w307 _]
    frame Disabled {
      n215 = while {
        tunnel: [w311] -> _
        tunnel: w307 -> [w311]
        stop <- FALSE stop-if-true
        # "ENCODER TESTING - 10ms"
        n216 = Unbundle By Name(w311) -> ("MotorControlDevRef"=w312:T6)
        n217 = case shown="True" FALSE {
          tunnel: w312 -> [_ w319]
          frame False {
          }
          frame True {
            n218 = call <vilib>:"WPI_CANTalonSRX_SetSensorPosition.vi"("New Sensor Position"=0.0, "CAN Talon SRX Ref"=w319) -> ()  [unwired: 8 in, 2 out]
          }
        }
        n219 = call <vilib>:"WPI_CANTalonSRX_GetStatus.vi"("Clear Sticky Faults"=FALSE, "CAN Talon SRX Ref"=w312) -> ("Talon SRX Status"=w315:T19)  [unwired: 7 in, 2 out]
        n220 = Unbundle By Name(w315) -> ("Sensor Position"=→"Sensor Position":dbl)
        n221 = Unbundle By Name(w315) -> ("Closed Loop Error"=→"Closed Loop Error":dbl)
        n222 = call <vilib>:"WPI_MotorControlSetOutput.vi"("Output"="Expected position", "MotorControlDevRef"=w312) -> ()  [unwired: 7 in, 3 out]
        n223 = Wait (ms)(milliseconds to wait=u32 10) -> ()  [unwired: 1 out]
      }
    }
    frame Enabled {
    }
  }
  n224 = while {
    shift-right: [w322] -> _
    shift-left: w1 -> [w323]
    stop <- FALSE stop-if-true
    n225 = case shown="True" "Forklift Method" {
      tunnel: w323 -> [w328 w356]
      tunnel: [w328 w356] -> w322
      frame False {
        (unwired) FALSE
        # "Low mode"
        # "Intake mode"
        # "Shooter"
        # "Right"
        # "Both"
        # "Left"
        # "Right Forklift"
        # "Left Forklift"
        # "Shooter"
        # "FORKLIFT HOLD - 10ms"
        n226 = global read "Robot Global Data.vi" "Joystick Butt 3"() -> (w327:bool)
        n227 = global read "Robot Global Data.vi" "Joystick Butt 11"() -> (w335:bool)
        n228 = global read "Robot Global Data.vi" "Joystick Butt 4"() -> (w330:bool)
        n229 = global read "Robot Global Data.vi" "Joystick Butt 8"() -> (w331:bool)
        "Intake Mode" <- w331
        n230 = global read "Robot Global Data.vi" "Joystick Butt 7"() -> (w325:bool)
        "Low Mode" <- w325
        n231 = global read "Robot Global Data.vi" "Joystick Butt 12"() -> (w333:bool)
        n232 = Or(x=w331, y=w325) -> (x .or. y?=w324:bool)
        n233 = Or(x=w330, y=w324) -> (x .or. y?=w329:bool)
        n234 = Or(x=w327, y=w325) -> (x .or. y?=w326:bool)
        n235 = Or(x=w335, y=w329) -> (x .or. y?=w334:bool)
        n236 = Or(x=w329, y=w333) -> (x .or. y?=w332:bool)
        n237 = Select(t=WPI_SolenoidValue."Forward" ("Value"), s=w326, f=WPI_SolenoidValue."Reverse" ("Value")) -> (s? t:f=w344:T20)
        n238 = Select(t=WPI_SolenoidValue."Forward" ("Value"), s=w332, f=WPI_SolenoidValue."Reverse" ("Value")) -> (s? t:f=w338:T20)
        n239 = Select(t=WPI_SolenoidValue."Forward" ("Value"), s=w334, f=WPI_SolenoidValue."Reverse" ("Value")) -> (s? t:f=w337:T20)
        n240 = Unbundle By Name(w328) -> ("SolenoidDevRef"=w345:T1)
        n241 = call-poly <vilib>:"WPI_SolenoidSet.vi"("Value"=w344, "SolenoidDevRef"=w345) -> ()  [unwired: 8 in, 2 out]
        n242 = Unbundle By Name(w328) -> ("SolenoidDevRef"=w340:T1)
        n243 = call-poly <vilib>:"WPI_SolenoidSet.vi"("Value"=w337, "SolenoidDevRef"=w340) -> ()  [unwired: 8 in, 2 out]
        n244 = Unbundle By Name(w328) -> ("SolenoidDevRef"=w339:T1)
        n245 = call-poly <vilib>:"WPI_SolenoidSet.vi"("Value"=w338, "SolenoidDevRef"=w339) -> ()  [unwired: 8 in, 2 out]
        n246 = Wait (ms)(milliseconds to wait=u32 10) -> ()  [unwired: 1 out]
      }
      frame True {
        (unwired) FALSE
        # "Low mode"
        # "Intake mode"
        # "Right Down"
        # "Right Up"
        # "Left Down"
        # "Left Up"
        # "Both Down"
        # "Shooter"
        # "Both Up"
        # "SH"
        # "Shooter"
        # "RD"
        # "RU"
        # "LD"
        # "LU"
        # "Left FL"
        # "Right FL"
        # "FORKLIFT TOGGLE - 10ms"
        n247 = global read "Robot Global Data.vi" "Joystick Butt 3"() -> (w354:bool)
        n248 = global read "Robot Global Data.vi" "Joystick Butt 10"() -> (w360:bool)
        n249 = global read "Robot Global Data.vi" "Joystick Butt 4"() -> (w359:bool)
        n250 = global read "Robot Global Data.vi" "Joystick Butt 8"() -> (w358:bool)
        n251 = local write "Intake Mode"(w358) -> ()
        n252 = global read "Robot Global Data.vi" "Joystick Butt 7"() -> (w349:bool)
        n253 = local write "Low Mode"(w349) -> ()
        n254 = global read "Robot Global Data.vi" "Joystick Butt 6"() -> (w364:bool)
        n255 = global read "Robot Global Data.vi" "Joystick Butt 11"() -> (w362:bool)
        n256 = global read "Robot Global Data.vi" "Joystick Butt 12"() -> (w363:bool)
        n257 = global read "Robot Global Data.vi" "Joystick Butt 9"() -> (w361:bool)
        n258 = Or(x=w358, y=w349) -> (x .or. y?=w350:bool)
        n259 = Or(x=w359, y=w350) -> (x .or. y?=w355:bool)
        n260 = Or(x=w354, y=w349) -> (x .or. y?=w353:bool)
        n261 = Or(x=w355, y=w362) -> (x .or. y?=w382:bool)
        "RU before" <- w382
        n262 = Or(x=w364, y=w363) -> (x .or. y?=w383:bool)
        "RD before" <- w383
        n263 = Or(x=w364, y=w360) -> (x .or. y?=w374:bool)
        "LD before" <- w374
        n264 = Or(x=w355, y=w361) -> (x .or. y?=w375:bool)
        "LU before" <- w375
        n265 = Not(x=w383) -> (.not. x?=w380:bool)
        n266 = Not(x=w374) -> (.not. x?=w377:bool)
        n267 = Not(x=w353) -> (.not. x?=w368:bool)
        n268 = feedback #1() -> (w381:bool)  [unwired: 1 in]
        n269 = And(x=w380, y=w381) -> (x .and. y?=w379:bool)
        n270 = feedback #2() -> (w378:bool)  [unwired: 1 in]
        n271 = And(x=w377, y=w378) -> (x .and. y?=w376:bool)
        n272 = Or(x=w382, y=w379) -> (x .or. y?=w352:bool)
        "R after" <- w352
        n273 = feedback-in #1(w352) -> ()
        n274 = feedback #3() -> (w365:bool)  [unwired: 1 in]
        n275 = Not(x=w365) -> (.not. x?=w369:bool)
        n276 = And(x=w368, y=w365) -> (x .and. y?=w367:bool)
        n277 = And(x=w353, y=w369) -> (x .and. y?=w366:bool)
        n278 = Or(x=w367, y=w366) -> (x .or. y?=w357:bool)
        n279 = feedback-in #3(w357) -> ()
        n280 = Or(x=w375, y=w376) -> (x .or. y?=w351:bool)
        "L after" <- w351
        n281 = feedback-in #2(w351) -> ()
        n282 = Unbundle By Name(w356) -> ("SolenoidDevRef"=w373:T1)
        n283 = Select(t=WPI_SolenoidValue."Forward" ("Value"), s=w357, f=WPI_SolenoidValue."Reverse" ("Value")) -> (s? t:f=w370:T20)
        n284 = call-poly <vilib>:"WPI_SolenoidSet.vi"("Value"=w370, "SolenoidDevRef"=w373) -> ()  [unwired: 8 in, 2 out]
        n285 = Unbundle By Name(w356) -> ("SolenoidDevRef"=w388:T1)
        n286 = Select(t=WPI_SolenoidValue."Forward" ("Value"), s=w351, f=WPI_SolenoidValue."Reverse" ("Value")) -> (s? t:f=w389:T20)
        n287 = call-poly <vilib>:"WPI_SolenoidSet.vi"("Value"=w389, "SolenoidDevRef"=w388) -> ()  [unwired: 8 in, 2 out]
        n288 = Unbundle By Name(w356) -> ("SolenoidDevRef"=w387:T1)
        n289 = Select(t=WPI_SolenoidValue."Forward" ("Value"), s=w352, f=WPI_SolenoidValue."Reverse" ("Value")) -> (s? t:f=w385:T20)
        n290 = call-poly <vilib>:"WPI_SolenoidSet.vi"("Value"=w385, "SolenoidDevRef"=w387) -> ()  [unwired: 8 in, 2 out]
        n291 = Wait (ms)(milliseconds to wait=u32 10) -> ()  [unwired: 1 out]
      }
    }
  }
  n292 = while {
    shift-right: [w400] -> _
    shift-left: w1 -> [w400]
    shift-right: [w403] -> _
    shift-left: _ -> [w401]
    stop <- FALSE stop-if-true
    # "LIGHTS - 10ms"
    n293 = Wait (ms)(milliseconds to wait=u32 10) -> ()  [unwired: 1 out]
    n294 = global read "Robot Global Data.vi" "Joystick Y"() -> (w399:dbl)
    n295 = Greater?(x=w399, y=0.1) -> (0:w408:bool)
    n296 = Less?(x=w399, y=-0.1) -> (x < y?=w409:bool)
    n297 = global read "Robot Global Data.vi" "Drive Mode"() -> (w411:bool)
    n298 = Or(x=w408, y=w409) -> (x .or. y?=w407:bool)
    n299 = Select(t=33.0, s=w408, f=34.0) -> (s? t:f=w412:dbl)
    n300 = Not(x=w407) -> (.not. x?=w406:bool)
    n301 = local read "Shoot Sequence Position"() -> (w398:dbl)
    n302 = Equal?(x=w398, y=1.0) -> (x = y?=w396:bool)
    n303 = Select(t=39.0, s=w396, f=40.0) -> (s? t:f=w393:dbl)
    n304 = Select(t=w393, s=w411, f=w412) -> (s? t:f=w405:dbl)
    n305 = Select(t=w405, s=w406, f=43.0) -> (s? t:f=w403:dbl)
    n306 = Not Equal?(x=w403, y=w401) -> (x != y?=w402:bool)
    n307 = case shown="True" w402 {
      tunnel: w403 -> [_ w419]
      tunnel: w400 -> [_ w418]
      frame False {
      }
      frame True {
        n308 = Unbundle By Name(w418) -> ("I2CDevRef"=w420:T13)
        n309 = call <vilib>:"WPI_I2CWrite.vi"("I2CRegister"=w419, "I2CDevRef"=w420) -> ()  [unwired: 8 in, 2 out]
      }
    }
  }
